vi "CMD_Harvest.vi"(1 "Line":string) -> (0 "Done":bool)   [LabVIEW 2014]
panel:
  in  "Parameters":i32[](array[numeric])=[1, 1, 1, 1]
  in  "Subcommands":string[](array[string])=["motor", "at", "for", "until"]
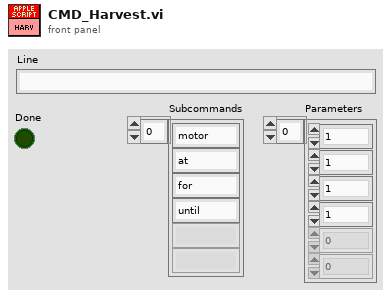
[diagram p1: front panel]
types:
  T1 = typedef "WPI_MotorControlDeviceRef.ctl" = cluster{"DeviceStatus":errorcluster, "Type":T2, "PWM":cluster{"Controller":T3, "PWM Channel":T4, "DeadBand":T5}, "CAN":cluster{"Device Number":u8, "Control Mode":T6, "Semaphore":T7, "Max Vout":dbl, "TalonSRX Control Mode":T8}, "Invert":bool, "TransformRef":T9, "InvTransformRef":T9}
  T2 = typedef "WPI_MotorControlType.ctl" = enum16{"PWM", "CAN", "CANTalonSRX"}
  T3 = typedef "FPGA_TypedefDigitalModule.ctl" = enum16{"Controller 1"}
  T4 = typedef "FPGA_DIOPWMChannel.ctl" = enum8{"PWM 0", "PWM 1", "PWM 2", "PWM 3", "PWM 4", "PWM 5", "PWM 6", "PWM 7", "PWM 8", "PWM 9", "PWM MXP 0", "PWM MXP 1", "PWM MXP 2", "PWM MXP 3", "PWM MXP 4", "PWM MXP 5", "PWM MXP 6", "PWM MXP 7", "PWM MXP 8", "PWM MXP 9", "Invalid"}
  T5 = typedef "WPI_PWMDeadband.ctl" = cluster{"Name":string, "maxPositivePwm":i32, "minPositivePwm":i32, "centerPwm":i32, "maxNegativePwm":i32, "minNegativePwm":i32, "angularRange":u16}
  T6 = typedef "WPI_CANJaguar_ControlMode.ctl" = enum8{"Percent VBus", "Current", "Speed", "Position", "Voltage"}
  T7 = typedef "Semaphore RefNum" = refnum<k1>
  T8 = typedef "WPI_CANTalonSRX_APIControlMode.ctl" = enum8{"Percent VBus", "Speed", "Position", "Slave", "Unchanged / Invalid"}
  T9 = typedef "WPI_PWMTransform_ConPane.ctl" = refnum<vi>
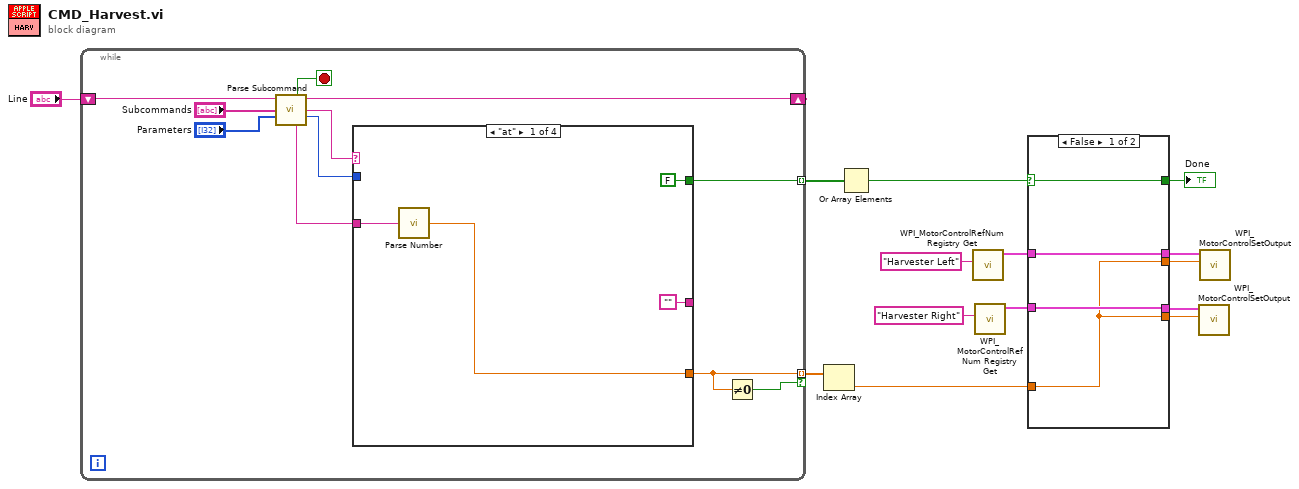
[diagram p0: block diagram]
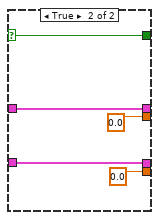
[diagram p2: hidden frame]
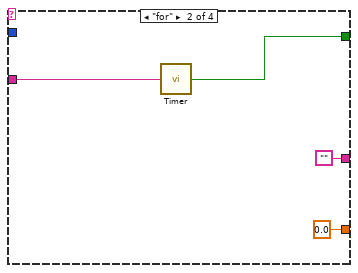
[diagram p3: hidden frame]
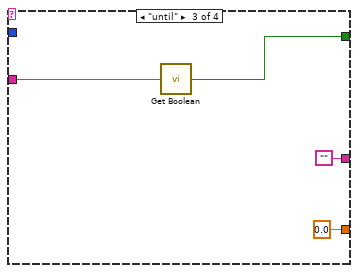
[diagram p4: hidden frame]
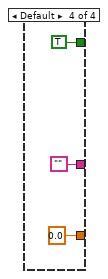
[diagram p5: hidden frame]
diagram:
  n1 = while {
    shift-right: [w22] -> _
    shift-left: "Line" -> [w25]
    tunnel: [w17] -> w13 mode=indexing
    tunnel: [w16] -> w12 mode=indexing if=w15
    stop <- w21 stop-if-true
    n2 = call "Parse Subcommand.vi"("Text In"=w25, "Subcommands"="Subcommands", "Parameters"="Parameters") -> ("Done"=w21:bool, "Text Out"=w22:string, "Subcommand"=w20:string, "# of Parameters"=w19:i32, "Parameter 1"=w18:string)  [unwired: 6 in, 2 out]
    n3 = case shown="\"at\"" w20 {
      tunnel: w19 -> [_ _ _ _]
      tunnel: w18 -> [w29 w33 w37 _]
      tunnel: [FALSE ("Value") w30 w34 TRUE ("Value")] -> w17
      tunnel: ["" "" "" ""] -> _
      tunnel: [w26 0.0 ("Number") 0.0 ("Number") 0.0 ("Number")] -> w16
      frame "at" {
        n4 = call "Parse Number.vi"("String"=w29) -> ("Number"=w26:dbl)
      }
      frame "for" {
        n5 = call "Timer.vi"("Seconds (string)"=w33) -> ("Done"=w30:bool)
      }
      frame "until" {
        n6 = call "Get Boolean.vi"("Name"=w37) -> ("Value"=w34:bool)
      }
      frame Default {
      }
    }
    n7 = Not Equal To 0?(x=w16) -> (x != 0?=w15:bool)
  }
  n8 = Index Array(array=w12) -> (element=w7:dbl)  [unwired: 1 in]
  n9 = Or Array Elements(Boolean array=w13) -> (logical OR=w11:bool)
  n10 = call <vilib>:"WPI_MotorControlRefNum Registry Get.vi"("refnum name"="Harvester Left") -> ("MotorControlDevRef"=w3:T1)  [unwired: 9 in, 1 out]
  n11 = call <vilib>:"WPI_MotorControlRefNum Registry Get.vi"("refnum name"="Harvester Right") -> ("MotorControlDevRef"=w9:T1)  [unwired: 9 in, 1 out]
  n12 = case shown="False" w11 {
    selector: w11 -> [w44 w49]
    tunnel: [w44 w49] -> w10
    tunnel: w9 -> [w43 w48]
    tunnel: [w43 w48] -> w8
    tunnel: w7 -> [w42 _]
    tunnel: [w42 0.0] -> w6
    tunnel: [w42 0.0] -> w1
    tunnel: w3 -> [w41 w45]
    tunnel: [w41 w45] -> w2
    frame False {
    }
    frame True {
    }
  }
  "Done" <- w10
  n13 = call <vilib>:"WPI_MotorControlSetOutput.vi"("Output"=w6, "MotorControlDevRef"=w8) -> ()  [unwired: 7 in, 3 out]
  n14 = call <vilib>:"WPI_MotorControlSetOutput.vi"("Output"=w1, "MotorControlDevRef"=w2) -> ()  [unwired: 7 in, 3 out]
